vi "DriverStation Set Op Mode Options.vi"(8 "error in (no error)":errorcluster, 11 "opModes":T1(array[cluster])) -> (0 "error out":errorcluster)   [LabVIEW 2026, in "MrcLib.lvlib"]
doc: "Lower level VI used to update all OpModes to DS."
uses:
  MrcLib.lvlib
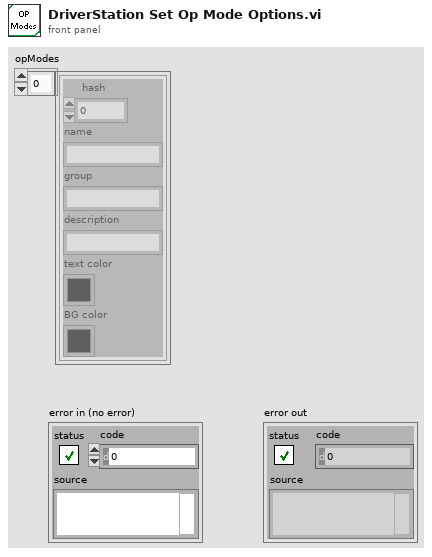
[diagram p1: front panel]
types:
  T1 = cluster{"hash":u64, "name":string, "group":string, "description":string, "text color":u32, "BG color":u32}[]
  T2 = cluster{u8, "unsigned byte array":cluster{"unsigned byte array[0]":u8, "unsigned byte array[1]":u8, "unsigned byte array[2]":u8, "unsigned byte array[3]":u8, "unsigned byte array[4]":u8, "unsigned byte array[5]":u8, "unsigned byte array[6]":u8, "unsigned byte array[7]":u8, "unsigned byte array[8]":u8, "unsigned byte array[9]":u8, "unsigned byte array[10]":u8, "unsigned byte array[11]":u8, "unsigned byte array[12]":u8, "unsigned byte array[13]":u8, "unsigned byte array[14]":u8, "unsigned byte array[15]":u8, "unsigned byte array[16]":u8, "unsigned byte array[17]":u8, "unsigned byte array[18]":u8, "unsigned byte array[19]":u8, "unsigned byte array[20]":u8, "unsigned byte array[21]":u8, "unsigned byte array[22]":u8, "unsigned byte array[23]":u8, "unsigned byte array[24]":u8, "unsigned byte array[25]":u8, "unsigned byte array[26]":u8, "unsigned byte array[27]":u8, "unsigned byte array[28]":u8, "unsigned byte array[29]":u8, "unsigned byte array[30]":u8, "unsigned byte array[31]":u8, "unsigned byte array[32]":u8, "unsigned byte array[33]":u8, "unsigned byte array[34]":u8, "unsigned byte array[35]":u8, "unsigned byte array[36]":u8, "unsigned byte array[37]":u8, "unsigned byte array[38]":u8, "unsigned byte array[39]":u8, "unsigned byte array[40]":u8, "unsigned byte array[41]":u8, "unsigned byte array[42]":u8, "unsigned byte array[43]":u8, "unsigned byte array[44]":u8, "unsigned byte array[45]":u8, "unsigned byte array[46]":u8, "unsigned byte array[47]":u8, "unsigned byte array[48]":u8, "unsigned byte array[49]":u8, "unsigned byte array[50]":u8, "unsigned byte array[51]":u8, "unsigned byte array[52]":u8, "unsigned byte array[53]":u8, "unsigned byte array[54]":u8, "unsigned byte array[55]":u8, "unsigned byte array[56]":u8, "unsigned byte array[57]":u8, "unsigned byte array[58]":u8, "unsigned byte array[59]":u8, "unsigned byte array[60]":u8, "unsigned byte array[61]":u8, "unsigned byte array[62]":u8, "unsigned byte array[63]":u8}}
  T3 = cluster{"hash":u64, "str64":cluster{u8, "unsigned byte array":cluster{"unsigned byte array[0]":u8, "unsigned byte array[1]":u8, "unsigned byte array[2]":u8, "unsigned byte array[3]":u8, "unsigned byte array[4]":u8, "unsigned byte array[5]":u8, "unsigned byte array[6]":u8, "unsigned byte array[7]":u8, "unsigned byte array[8]":u8, "unsigned byte array[9]":u8, "unsigned byte array[10]":u8, "unsigned byte array[11]":u8, "unsigned byte array[12]":u8, "unsigned byte array[13]":u8, "unsigned byte array[14]":u8, "unsigned byte array[15]":u8, "unsigned byte array[16]":u8, "unsigned byte array[17]":u8, "unsigned byte array[18]":u8, "unsigned byte array[19]":u8, "unsigned byte array[20]":u8, "unsigned byte array[21]":u8, "unsigned byte array[22]":u8, "unsigned byte array[23]":u8, "unsigned byte array[24]":u8, "unsigned byte array[25]":u8, "unsigned byte array[26]":u8, "unsigned byte array[27]":u8, "unsigned byte array[28]":u8, "unsigned byte array[29]":u8, "unsigned byte array[30]":u8, "unsigned byte array[31]":u8, "unsigned byte array[32]":u8, "unsigned byte array[33]":u8, "unsigned byte array[34]":u8, "unsigned byte array[35]":u8, "unsigned byte array[36]":u8, "unsigned byte array[37]":u8, "unsigned byte array[38]":u8, "unsigned byte array[39]":u8, "unsigned byte array[40]":u8, "unsigned byte array[41]":u8, "unsigned byte array[42]":u8, "unsigned byte array[43]":u8, "unsigned byte array[44]":u8, "unsigned byte array[45]":u8, "unsigned byte array[46]":u8, "unsigned byte array[47]":u8, "unsigned byte array[48]":u8, "unsigned byte array[49]":u8, "unsigned byte array[50]":u8, "unsigned byte array[51]":u8, "unsigned byte array[52]":u8, "unsigned byte array[53]":u8, "unsigned byte array[54]":u8, "unsigned byte array[55]":u8, "unsigned byte array[56]":u8, "unsigned byte array[57]":u8, "unsigned byte array[58]":u8, "unsigned byte array[59]":u8, "unsigned byte array[60]":u8, "unsigned byte array[61]":u8, "unsigned byte array[62]":u8, "unsigned byte array[63]":u8}}, "str64":cluster{u8, "unsigned byte array":cluster{"unsigned byte array[0]":u8, "unsigned byte array[1]":u8, "unsigned byte array[2]":u8, "unsigned byte array[3]":u8, "unsigned byte array[4]":u8, "unsigned byte array[5]":u8, "unsigned byte array[6]":u8, "unsigned byte array[7]":u8, "unsigned byte array[8]":u8, "unsigned byte array[9]":u8, "unsigned byte array[10]":u8, "unsigned byte array[11]":u8, "unsigned byte array[12]":u8, "unsigned byte array[13]":u8, "unsigned byte array[14]":u8, "unsigned byte array[15]":u8, "unsigned byte array[16]":u8, "unsigned byte array[17]":u8, "unsigned byte array[18]":u8, "unsigned byte array[19]":u8, "unsigned byte array[20]":u8, "unsigned byte array[21]":u8, "unsigned byte array[22]":u8, "unsigned byte array[23]":u8, "unsigned byte array[24]":u8, "unsigned byte array[25]":u8, "unsigned byte array[26]":u8, "unsigned byte array[27]":u8, "unsigned byte array[28]":u8, "unsigned byte array[29]":u8, "unsigned byte array[30]":u8, "unsigned byte array[31]":u8, "unsigned byte array[32]":u8, "unsigned byte array[33]":u8, "unsigned byte array[34]":u8, "unsigned byte array[35]":u8, "unsigned byte array[36]":u8, "unsigned byte array[37]":u8, "unsigned byte array[38]":u8, "unsigned byte array[39]":u8, "unsigned byte array[40]":u8, "unsigned byte array[41]":u8, "unsigned byte array[42]":u8, "unsigned byte array[43]":u8, "unsigned byte array[44]":u8, "unsigned byte array[45]":u8, "unsigned byte array[46]":u8, "unsigned byte array[47]":u8, "unsigned byte array[48]":u8, "unsigned byte array[49]":u8, "unsigned byte array[50]":u8, "unsigned byte array[51]":u8, "unsigned byte array[52]":u8, "unsigned byte array[53]":u8, "unsigned byte array[54]":u8, "unsigned byte array[55]":u8, "unsigned byte array[56]":u8, "unsigned byte array[57]":u8, "unsigned byte array[58]":u8, "unsigned byte array[59]":u8, "unsigned byte array[60]":u8, "unsigned byte array[61]":u8, "unsigned byte array[62]":u8, "unsigned byte array[63]":u8}}, "str64":cluster{u8, "unsigned byte array":cluster{"unsigned byte array[0]":u8, "unsigned byte array[1]":u8, "unsigned byte array[2]":u8, "unsigned byte array[3]":u8, "unsigned byte array[4]":u8, "unsigned byte array[5]":u8, "unsigned byte array[6]":u8, "unsigned byte array[7]":u8, "unsigned byte array[8]":u8, "unsigned byte array[9]":u8, "unsigned byte array[10]":u8, "unsigned byte array[11]":u8, "unsigned byte array[12]":u8, "unsigned byte array[13]":u8, "unsigned byte array[14]":u8, "unsigned byte array[15]":u8, "unsigned byte array[16]":u8, "unsigned byte array[17]":u8, "unsigned byte array[18]":u8, "unsigned byte array[19]":u8, "unsigned byte array[20]":u8, "unsigned byte array[21]":u8, "unsigned byte array[22]":u8, "unsigned byte array[23]":u8, "unsigned byte array[24]":u8, "unsigned byte array[25]":u8, "unsigned byte array[26]":u8, "unsigned byte array[27]":u8, "unsigned byte array[28]":u8, "unsigned byte array[29]":u8, "unsigned byte array[30]":u8, "unsigned byte array[31]":u8, "unsigned byte array[32]":u8, "unsigned byte array[33]":u8, "unsigned byte array[34]":u8, "unsigned byte array[35]":u8, "unsigned byte array[36]":u8, "unsigned byte array[37]":u8, "unsigned byte array[38]":u8, "unsigned byte array[39]":u8, "unsigned byte array[40]":u8, "unsigned byte array[41]":u8, "unsigned byte array[42]":u8, "unsigned byte array[43]":u8, "unsigned byte array[44]":u8, "unsigned byte array[45]":u8, "unsigned byte array[46]":u8, "unsigned byte array[47]":u8, "unsigned byte array[48]":u8, "unsigned byte array[49]":u8, "unsigned byte array[50]":u8, "unsigned byte array[51]":u8, "unsigned byte array[52]":u8, "unsigned byte array[53]":u8, "unsigned byte array[54]":u8, "unsigned byte array[55]":u8, "unsigned byte array[56]":u8, "unsigned byte array[57]":u8, "unsigned byte array[58]":u8, "unsigned byte array[59]":u8, "unsigned byte array[60]":u8, "unsigned byte array[61]":u8, "unsigned byte array[62]":u8, "unsigned byte array[63]":u8}}, "text color":u32, "BG color":u32}
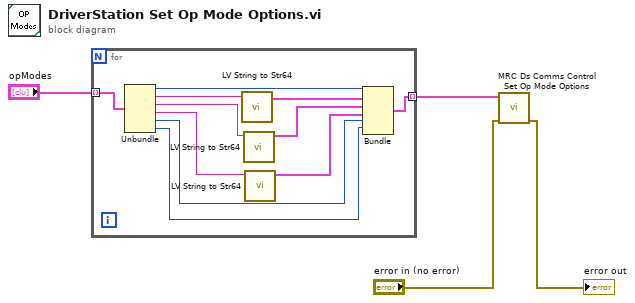
[diagram p0: block diagram]
diagram:
  n1 = for {
    tunnel: "opModes" -> [w15] mode=indexing
    tunnel: [w14] -> w3 mode=indexing
    n2 = Unbundle(w15) -> ("hash"=w13:u64, "name"=w10:string, "group"=w8:string, "description"=w6:string, "text color"=w11:u32, "BG color"=w12:u32)
    n3 = call "LV String to Str64.vi"("string"=w10) -> ("str64"=w9:T2)  [unwired: 10 in]
    n4 = call "LV String to Str64.vi"("string"=w8) -> ("str64"=w7:T2)  [unwired: 10 in]
    n5 = call "LV String to Str64.vi"("string"=w6) -> ("str64"=w5:T2)  [unwired: 10 in]
    n6 = Bundle("hash"=w13, "str64"=w9, "str64"=w7, "str64"=w5, "text color"=w11, "BG color"=w12) -> (w14:T3)  [unwired: 1 in]
  }
  n7 = call "MRC Ds Comms Control Set Op Mode Options.vi"("error in (no error)"="error in (no error)", "opModes"=w3) -> ("error out"=→"error out":errorcluster)  [unwired: 9 in]
